vi "Tell Reply.vi"(4 "Priority":bool, 6 "Teller":refnum<class "Teller.lvclass">, 7 "Actor in":refnum<class "Actor.lvclass">, 9 "Error":errorcluster, 10 "Actor":refnum<class "Actor.lvclass">) -> (0 "Error out":errorcluster)   [LabVIEW 2025, in "jettl.lvlib" / "Terminate Msg.lvlib"]
uses:
  Terminate Msg.lvlib
  Terminate Msg/Terminate Msg.lvclass
  C:/git/jettl/src/jettl/jettl/Terminate Msg/Finish Msg/Terminate Msg.lvclass
  C:/git/jettl/src/jettl/jettl/Msg/Msg.lvclass
  Actor/Actor/Actor.lvclass
  Teller/Teller/Teller.lvclass
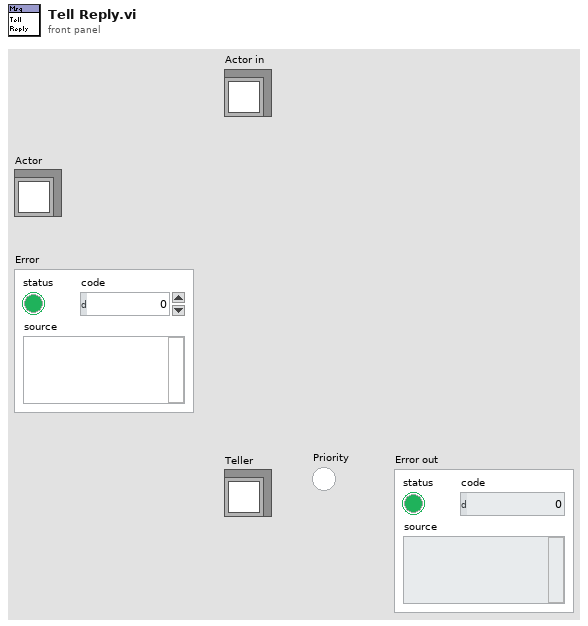
[diagram p1: front panel]
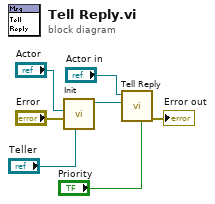
[diagram p0: block diagram]
diagram:
  n1 = call "Init.vi"("Teller"="Teller", "Error"="Error", "Actor"="Actor") -> ("Terminate Msg out"=w3:refnum<class "Terminate Msg.lvclass">)  [unwired: 8 in]
  n2 = call-dynamic "Tell Reply.vi"("Priority"="Priority", "Msg"=w3, "Actor in"="Actor in") -> ("Error out"=→"Error out":errorcluster)  [unwired: 8 in]
